vi "Check External Interlocks.vi"(8 "error in (no error)":errorcluster, 11 "VISA resource name":refnum<visa-resource-name>) -> (0 "error out":errorcluster, 2 "External Interlocks State":u32(ring) items=["Disabled", "Enabled"], 3 "VISA resource name out":refnum<visa-resource-name>)   [LabVIEW 2022 SP3, in "MagnaDC.lvlib"]
uses:
  MagnaDC.lvlib
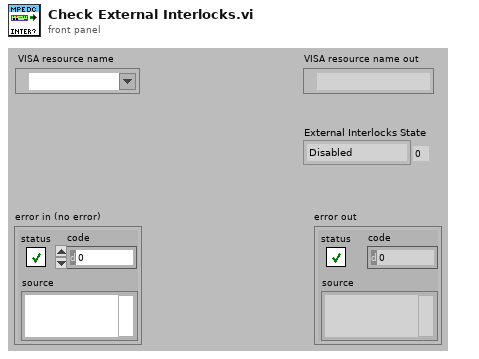
[diagram p1: front panel]
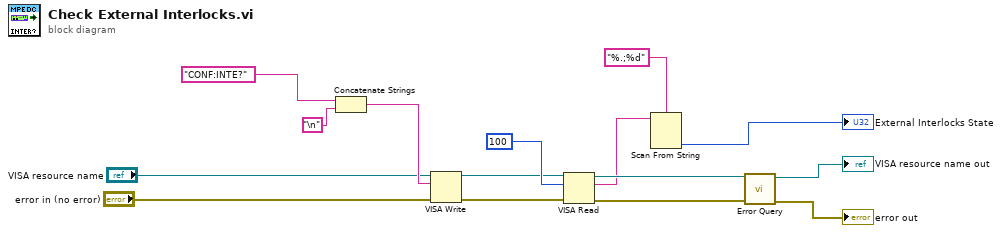
[diagram p0: block diagram]
diagram:
  n1 = Concatenate Strings("CONF:INTE?" ("Check Remote Sense Command"), "\n") -> (w8:string)
  n2 = VISA Write(VISA resource name="VISA resource name", write buffer=w8, error in (no error)="error in (no error)") -> (VISA resource name out=w5:refnum<visa-resource-name>, error out=w4:errorcluster)  [unwired: 1 out]
  n3 = VISA Read(VISA resource name=w5, byte count=u32 100, error in (no error)=w4) -> (VISA resource name out=w11:refnum<visa-resource-name>, read buffer=w2:string, error out=w10:errorcluster)  [unwired: 1 out]
  n4 = Scan From String(format string="%.;%d", input string=w2) -> (output 1=→"External Interlocks State":u32)  [unwired: 3 in, 3 out]
  n5 = call "Error Query.vi"("error in (no error)"=w10, "VISA resource name"=w11) -> ("error out"=→"error out":errorcluster, "VISA resource name out"=→"VISA resource name out":refnum<visa-resource-name>)  [unwired: 6 in, 2 out]
